vi "Encode Topic Subscriptions.vi"(10 "Topic Subscriptions":string[](array[string])) -> (2 "Length-Prefixed Field":u8[](array[numeric]))   [LabVIEW 2013, in "MQTT_Control_Packets.lvlib" / "UNSUBSCRIBE.lvclass"]
uses:
  UNSUBSCRIBE.lvclass
  ControlPacket/ControlPacket.lvclass
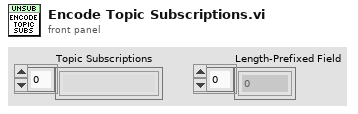
[diagram p1: front panel]
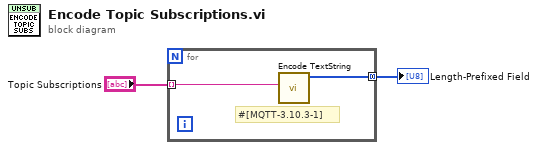
[diagram p0: block diagram]
diagram:
  n1 = for {
    tunnel: "Topic Subscriptions" -> [w4] mode=indexing
    tunnel: [w3] -> w2 mode=concatenating
    # "#[MQTT-3.10.3-1]"
    n2 = call "Encode TextString.vi"("Text String"=w4) -> ("Length-Prefixed Field"=w3:u8[])  [unwired: 10 in]
  }
  "Length-Prefixed Field" <- w2
